vi "Do.vi"(8 "error in (no error)":errorcluster, 10 "Actor in":refnum<class "Actor.lvclass">, 11 "Message":refnum<class "Message.lvclass">) -> (0 "error out":errorcluster, 2 "Actor out":refnum<class "Actor.lvclass">)   [LabVIEW 2020, in "Actor Framework.lvlib" / "Message.lvclass"]
doc: "(<B>Filename</B>: Actor Framework.lvlib:Message.lvclass:Do.vi)\n\nDefines what a message does when it is received by an actor. Generally, a message instructs an actor to invoke one of its methods. By default, this method does nothing. A child class must override it to define behavior."
uses:
  <vilib>/ActorFramework/Message/Message.lvclass
  <vilib>/ActorFramework/Actor/Actor.lvclass
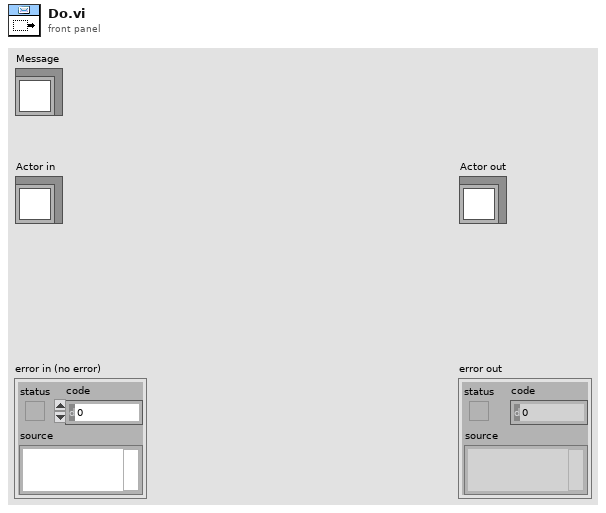
[diagram p1: front panel]
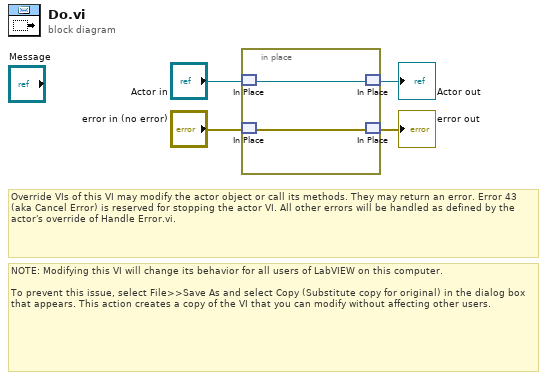
[diagram p0: block diagram]
diagram:
  # "NOTE: Modifying this VI will change its behavior for all users of LabVIEW on this computer.\n\nTo prevent this issue, select File>>Save As and select Copy (Substitute copy for original) in the dialog box that appears. This action creates a copy of the VI that you can modify without affecting other users."
  # "Override VIs of this VI may modify the actor object or call its methods. They may return an error. Error 43 (aka Cancel Error) is reserved for stopping the actor VI. All other errors will be handled as defined by the actor's override of Handle Error.vi."
  n1 = in-place {
    n2 = in-place-match #1("Actor in") -> (w5:refnum<class "Actor.lvclass">)
    n3 = in-place-match #2("error in (no error)") -> (w6:errorcluster)
    n4 = in-place-match #1(w5) -> (→"Actor out":refnum<class "Actor.lvclass">)
    n5 = in-place-match #2(w6) -> (→"error out":errorcluster)
  }
